vi "Server(UtilityMode).vi"() -> ()   [LabVIEW 2013, in "OPC UA Demo.lvlib"]
doc: "Demonstrates the use of the <B>OPC UA Server</B> VIs to programmatically create an OPC UA server."
uses:
  OPC UA Demo.lvlib
  <vilib>/OPCUA/server/Write Int32.vi
  <vilib>/OPCUA/server/Read Int32.vi
  <vilib>/OPCUA/NI OPC UA Server.lvlib
  OPCUA(Utility)/Server/OPCUA Server(UtilityMode).lvlib
panel:
  out "appended array":path[](array[path])
  out "Device.Node.Set Point":i32
  out "Device.Node":i32
  out "server endpoint URL":string
  out "error out":errorcluster
  in  "stop":bool
  # "Overview: Demonstrates the use of the OPC UA Server VIs to programmatically create an OPC UA server.\nRequirements: \n1. LabVIEW Datalogging and Supervisory Control Module or LabVIEW Real-Time Module\n2. (Real-Time Module) RT target\nInstructions:\nRun the VI."
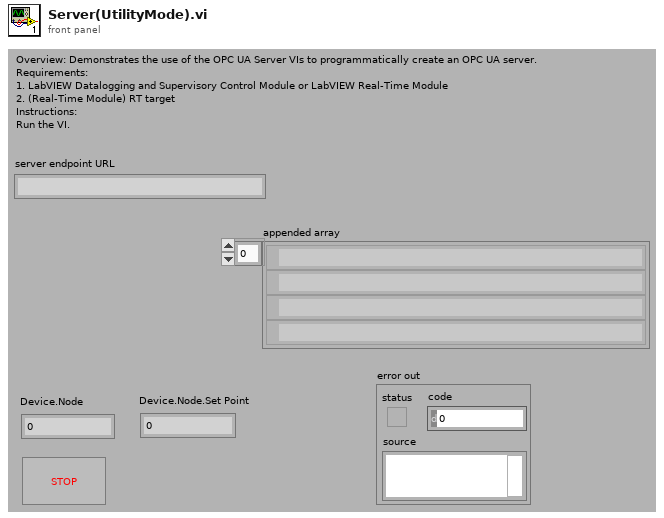
[diagram p1: front panel]
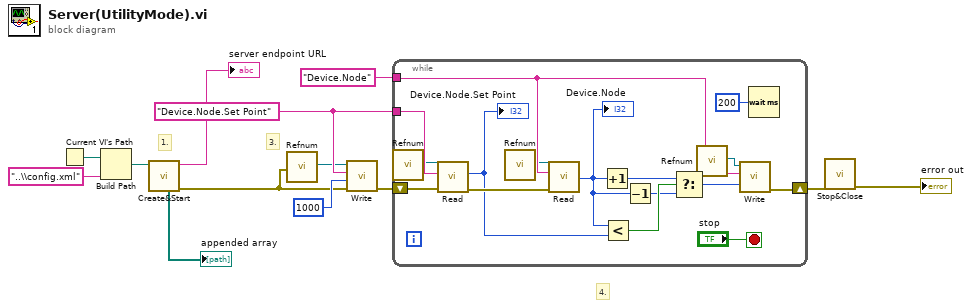
[diagram p0: block diagram]
diagram:
  w7 = "Device.Node.Set Point" ("property path")
  # "4."
  # "3."
  # "1."
  n1 = Current VI's Path() -> (path=w10:path)
  n2 = Build Path(base path=w10, name or relative path="..\\config.xml") -> (appended path=w8:path)
  n3 = call "Create&Start.vi"("XML config File Path"=w8) -> ("error out"=w2:errorcluster, "server endpoint URL"=→"server endpoint URL":string, "trusted client certfications"=→"appended array":path[])  [unwired: 7 in, 1 out]
  n4 = call "Refnum.vi"("error in (no error)"=w2) -> ("OPC UA server refnum"=w3:refnum<k21>)  [unwired: 17 in, 1 out]
  n5 = call-poly <vilib>:"Write.vi"("error in (no error)"=w2, "value"=1000, "node path"=w7, "OPC UA server refnum in"=w3) -> ("error out"=w12:errorcluster)  [unwired: 6 in, 1 out]
  n6 = while {
    tunnel: "Device.Node" ("item path") -> [w23]
    shift-right: [w26] -> w5
    shift-left: w12 -> [w28]
    tunnel: w7 -> [w25]
    stop <- "stop" stop-if-true
    n7 = call "Refnum.vi"() -> ("OPC UA server refnum"=w16:refnum<k21>)  [unwired: 18 in, 1 out]
    n8 = call-poly <vilib>:"Read.vi"("error in (no error)"=w28, "node path"=w25, "OPC UA server refnum in"=w16) -> ("error out"=w24:errorcluster, "value"=w22:i32)  [unwired: 4 in, 3 out]
    "Device.Node.Set Point" <- w22
    n9 = call "Refnum.vi"() -> ("OPC UA server refnum"=w15:refnum<k21>)  [unwired: 18 in, 1 out]
    n10 = call-poly <vilib>:"Read.vi"("error in (no error)"=w24, "node path"=w23, "OPC UA server refnum in"=w15) -> ("value"=w18:i32)  [unwired: 4 in, 4 out]
    "Device.Node" <- w18
    n11 = Increment(x=w18) -> (x+1=w20:i32)
    n12 = Less?(x=w18, y=w22) -> (x < y?=w21:bool)
    n13 = Decrement(x=w18) -> (x-1=w19:i32)
    n14 = Select(t=w20, s=w21, f=w19) -> (s? t:f=w17:i32)
    n15 = call "Refnum.vi"() -> ("OPC UA server refnum"=w14:refnum<k21>)  [unwired: 18 in, 1 out]
    n16 = call-poly <vilib>:"Write.vi"("value"=w17, "node path"=w23, "OPC UA server refnum in"=w14) -> ("error out"=w26:errorcluster)  [unwired: 7 in, 1 out]
    n17 = Wait (ms)(milliseconds to wait=u32 200) -> ()  [unwired: 1 out]
  }
  n18 = call "Stop&Close.vi"("error in (no error)"=w5) -> ("error out"=→"error out":errorcluster)  [unwired: 10 in]
